vi "ftp_client.vi"(5 "Computer IP":string="localhost", 6 "remote folder":string, 7 "password":string="stuff", 8 "error in (no error)":errorcluster, 10 "Files to move":path[](array[path]), 11 "files to transfer bin in":path) -> ()   [LabVIEW 2017, in "labview-standard-library.lvlib" / "file-transfer.lvlib"]
uses:
  file-transfer.lvlib
  <vilib>/FTP/NI_FTP.lvlib
panel:
  out "init connection error":errorcluster
  out "close reply":string
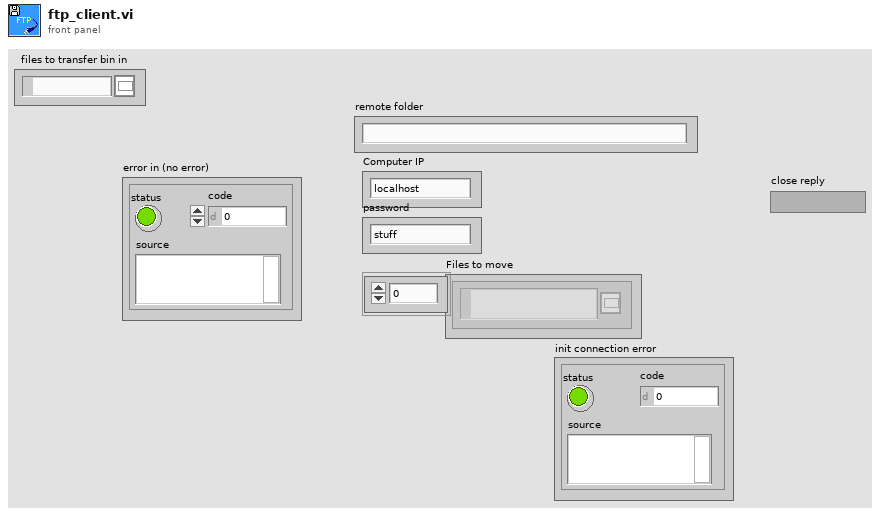
[diagram p1: front panel]
types:
  T1 = typedef "NI_FTP.lvlib/FTP Session.ctl" = refnum<k5>
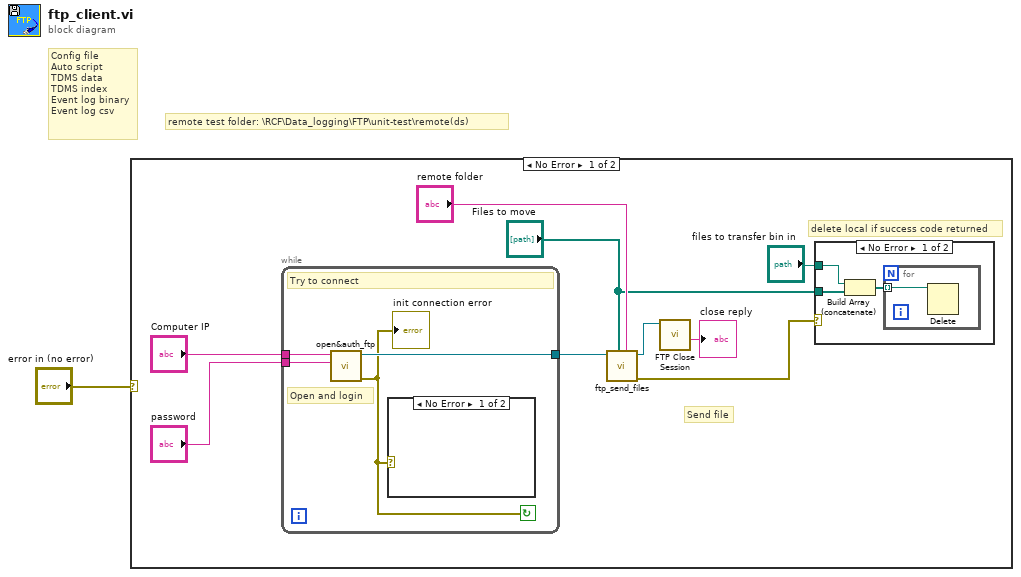
[diagram p0: block diagram]
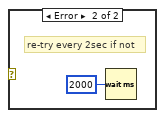
[diagram p3: hidden frame]
diagram:
  # "remote test folder: \\RCF\\Data_logging\\FTP\\unit-test\\remote(ds)"
  # "Config file\nAuto script\nTDMS data\nTDMS index\nEvent log binary\nEvent log csv"
  n1 = case shown="No Error" "error in (no error)" {
    frame No Error {
      # "delete local if success code returned"
      # "Send file"
      n2 = while {
        tunnel: "Computer IP" -> [w18]
        tunnel: "password" -> [w17]
        tunnel: [w16] -> w6
        stop <- w15 continue-if-true
        # "Open and login"
        # "Try to connect"
        n3 = call "open&auth_ftp.vi"("password"=w17, "Computer IP"=w18) -> ("error out"=w15:errorcluster, "TCP Network Connection out"=w16:T1)  [unwired: 8 in]
        "init connection error" <- w15
        n4 = case shown="No Error" w15 {
          frame No Error {
          }
          frame Error {
            # "re-try every 2sec if not"
            n5 = Wait (ms)(milliseconds to wait=u32 2000) -> ()  [unwired: 1 out]
          }
        }
      }
      n6 = call "ftp_send_files.vi"("remote folder"="remote folder", "Files to move"="Files to move", "ftp session in"=w6) -> ("error out"=w2:errorcluster, "ftp session out"=w5:T1)  [unwired: 7 in]
      n7 = call <vilib>:"FTP Close Session.vi"("ftp session"=w5) -> ("reply string"=→"close reply":string)  [unwired: 7 in, 3 out]
      n8 = case shown="No Error" w2 {
        tunnel: "files to transfer bin in" -> [w13 _]
        tunnel: "Files to move" -> [w12 _]
        frame No Error {
          n9 = Build Array (concatenate)(w13, w12) -> (w11:path[])
          n10 = for {
            tunnel: w11 -> [w14] mode=indexing
            n11 = Delete(path (use dialog)=w14) -> ()  [unwired: 4 in, 3 out]
          }
        }
        frame Error {
        }
      }
    }
    frame Error {
    }
  }
